vi "colourBg.vi"(8 "error in (no error)":errorcluster, 11 "ScriptEditorV2 in":refnum<class "ScriptEditorV2.lvclass">) -> (0 "error out":errorcluster, 3 "ScriptEditorV2 out":refnum<class "ScriptEditorV2.lvclass">)   [LabVIEW 2011, in "Views.lvlib" / "ScriptEditor.lvlib" / "ScriptEditorV2.lvclass"]
uses:
  ScriptEditorV2.lvclass
  ScriptEditorV2.lvclass/ScriptEditorV2.ctl
  Tools/DatabaseHelpers/DbConnection/DeviceDataBase/deviceDataBase.lvclass
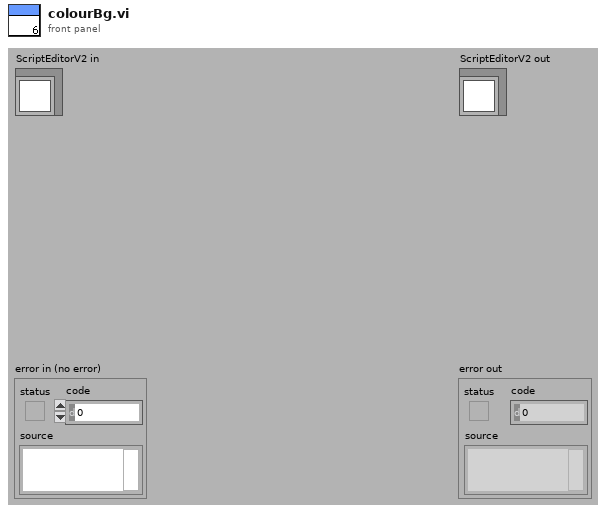
[diagram p1: front panel]
types:
  T1 = typedef "LVRowAndColumnUnsignedTypeDef.ctl" = cluster{"Row":u32, "Column":u32}
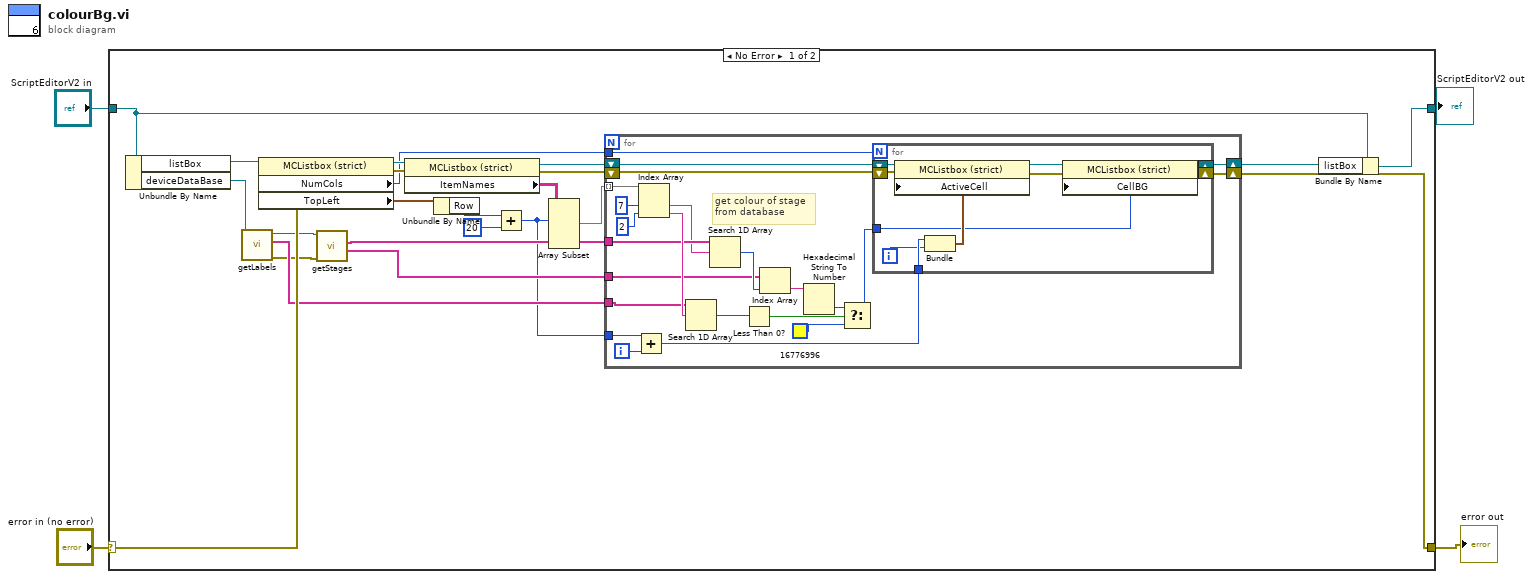
[diagram p0: block diagram]
diagram:
  n1 = case shown="No Error" "error in (no error)" {
    selector: "error in (no error)" -> [w24 w62]
    tunnel: [w17 w62] -> w3
    tunnel: [w20 w61] -> w1
    tunnel: "ScriptEditorV2 in" -> [w21 w61]
    frame No Error {
      n2 = Unbundle By Name(w21) -> ("listBox"=w23:refnum<vi>, "deviceDataBase"=w16:refnum<class "deviceDataBase.lvclass">)
      n3 = call "getLabels.vi"("deviceDataBase in"=w16) -> ("error out"=w13:errorcluster, "labels"=w15:string[], "deviceDataBase out"=w14:refnum<class "deviceDataBase.lvclass">)  [unwired: 8 in]
      n4 = property class="MCListbox (strict)"(reference=w23, error in=w24) -> (reference out=w26:refnum<vi>, error out=w25:errorcluster, "NumCols"=w22:u32, "TopLeft"=w10:T1)
      n5 = call "getStages.vi"("error in (no error)"=w13, "deviceDataBase in"=w14) -> ("colours"=w11:string[], "stages"=w12:string[])  [unwired: 6 in, 2 out]
      n6 = property class="MCListbox (strict)"(reference=w26, error in=w25) -> (reference out=w27:refnum<vi>, error out=w18:errorcluster, "ItemNames"=w9:string[][])
      n7 = Unbundle By Name(w10) -> ("Row"=w6:u32)
      n8 = Add(x=w6, y=20) -> (x+y=w5:u32)
      n9 = Array Subset(array=w9, index (row)=w5) -> (w8:string[][])  [unwired: 3 in]
      n10 = for {
        tunnel: w8 -> [w50] mode=indexing
        tunnel: w22 -> [w47]
        shift-right: [w46] -> w19
        shift-left: w27 -> [w48]
        shift-right: [w44] -> w17
        shift-left: w18 -> [w45]
        tunnel: w15 -> [w41]
        tunnel: w12 -> [w36]
        tunnel: w11 -> [w34]
        tunnel: w5 -> [w29]
        i -> [w30]
        # "get colour of stage\nfrom database"
        n11 = Add(x=w29, y=w30) -> (x+y=w28:u32)
        n12 = Index Array(array=w50, index #1=7, index #2=2) -> (element #1=w33:string, element #2=w42:string)
        n13 = Search 1D Array(1D array=w41, element=w42) -> (index of element=w37:i32)  [unwired: 1 in]
        n14 = Search 1D Array(1D array=w36, element=w33) -> (index of element=w35:i32)  [unwired: 1 in]
        n15 = Less Than 0?(x=w37) -> (x < 0?=w40:bool)
        n16 = Index Array(array=w34, index=w35) -> (element=w31:string)
        n17 = Hexadecimal String To Number(string=w31) -> (number=w32:u32)  [unwired: 2 in, 1 out]
        n18 = Select(t=w32, s=w40, f=u32 16776996) -> (s? t:f=w39:u32)
        n19 = for {
          N: w47 -> [_]
          tunnel: w28 -> [w52]
          shift-right: [w56] -> w46
          shift-left: w48 -> [w59]
          shift-right: [w54] -> w44
          shift-left: w45 -> [w55]
          tunnel: w39 -> [w53]
          i -> [w51]
          n20 = Bundle(w52, w51) -> (w57:cluster{u32, i32})  [unwired: 1 in]
          n21 = property class="MCListbox (strict)"(reference=w59, error in=w55, "ActiveCell"=w57) -> (reference out=w60:refnum<vi>, error out=w58:errorcluster)
          n22 = property class="MCListbox (strict)"(reference=w60, error in=w58, "CellBG"=w53) -> (reference out=w56:refnum<vi>, error out=w54:errorcluster)
        }
      }
      n23 = Bundle By Name(cluster=w21, "listBox"=w19) -> (w20:refnum<class "ScriptEditorV2.lvclass">)
    }
    frame Error {
    }
  }
  "error out" <- w3
  "ScriptEditorV2 out" <- w1
